vi "ConvertBase64StringToBytes.vi"(11 "Base64 string":string) -> (1 "error":bool, 3 "U8 array":u8[](array[numeric]))   [LabVIEW 2017]
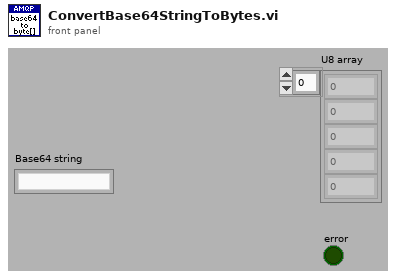
[diagram p1: front panel]
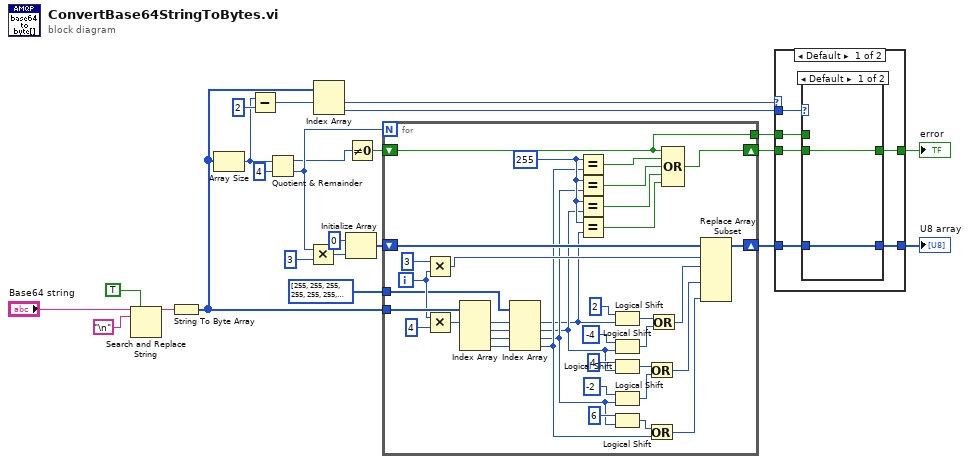
[diagram p0: block diagram]
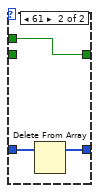
[diagram p2: hidden frame]
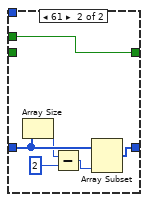
[diagram p3: hidden frame]
diagram:
  n1 = Search and Replace String(replace all?=TRUE ("replace all? (F)"), input string="Base64 string", search string="\n") -> (result string=w6:string)  [unwired: 1 in, 7 out]
  n2 = String To Byte Array(string=w6) -> (unsigned byte array=w9:u8[])
  n3 = Array Size(array=w9) -> (size(s)=w14:i32)
  n4 = Subtract(x=w14, y=2 ("x")) -> (x-y=w13:i32)
  n5 = Quotient & Remainder(x=w14, y=4) -> (x-y*floor(x/y)=w16:i32, floor(x/y)=w20:i32)
  n6 = Multiply(x=w20, y=3) -> (x*y=w19:i32)
  n7 = Index Array(array=w9, index #1=w13) -> (element #1=w12:u8, element #2=w11:u8)  [unwired: 1 in]
  n8 = Initialize Array(u8 0 ("Numeric"), w19) -> (w21:u8[])
  n9 = Not Equal To 0?(x=w16) -> (x != 0?=w8:bool)
  n10 = for {
    N: w20 -> [_]
    shift-right: [w57] -> w15
    shift-left: w21 -> [w58]
    tunnel: w9 -> [w61]
    tunnel: u8[] [255, 255, 255, 255, 255, 255, 255, 255, 255, 255, 255, 255, 255, 255, 255, 255, 255, 255, 255, 255, 255, 255, 255, 255, 255, 255, 255, 255, 255, 255, 255, 255, 255, 255, 255, 255, 255, 255, 255, 255, 255, 255, 255, 62, 255, 255, 255, 63, 52, 53, 54, 55, 56, 57, 58, 59, 60, 61, 255, 255, 255, 255, 255, 255, 255, 0, 1, 2, 3, 4, 5, 6, 7, 8, 9, 10, 11, 12, 13, 14, 15, 16, 17, 18, 19, 20, 21, 22, 23, 24, 25, 255, 255, 255, 255, 255, 255, 26, 27, 28, 29, 30, 31, 32, 33, 34, 35, 36, 37, 38, 39, 40, 41, 42, 43, 44, 45, 46, 47, 48, 49, 50, 51, 255, 255, 255, 255, 255, 255, 255, 255, 255, 255, 255, 255, 255, 255, 255, 255, 255, 255, 255, 255, 255, 255, 255, 255, 255, 255, 255, 255, 255, 255, 255, 255, 255, 255, 255, 255, 255, 255, 255, 255, 255, 255, 255, 255, 255, 255, 255, 255, 255, 255, 255, 255, 255, 255, 255, 255, 255, 255, 255, 255, 255, 255, 255, 255, 255, 255, 255, 255, 255, 255, 255, 255, 255, 255, 255, 255, 255, 255, 255, 255, 255, 255, 255, 255, 255, 255, 255, 255, 255, 255, 255, 255, 255, 255, 255, 255, 255, 255, 255, 255, 255, 255, 255, 255, 255, 255, 255, 255, 255, 255, 255, 255, 255, 255, 255, 255, 255, 255, 255, 255, 255, 255, 255, 255, 255, 255, 255, 255, 255, 255, 255, 255, 255] ("Array") -> [w43]
    shift-right: [w25] -> w2
    shift-left: w8 -> [w30]
    tunnel: [w30] -> w1
    i -> [w56]
    w35 = u8 255 ("x")
    n11 = Multiply(x=3, y=w56) -> (x*y=w54:i32)
    n12 = Multiply(x=w56, y=4 ("x")) -> (x*y=w59:i32)
    n13 = Index Array(array=w61, index #1=w59) -> (element #1=w42:u8, element #2=w41:u8, element #3=w40:u8, element #4=w39:u8)  [unwired: 3 in]
    n14 = Index Array(array=w43, index #1=w42, index #2=w41, index #3=w40, index #4=w39) -> (element #1=w26:u8, element #2=w27:u8, element #3=w28:u8, element #4=w29:u8)
    n15 = Equal?(x=w35, y=w29) -> (x = y?=w34:bool)
    n16 = Equal?(x=w35, y=w28) -> (x = y?=w33:bool)
    n17 = Equal?(x=w35, y=w27) -> (x = y?=w32:bool)
    n18 = Equal?(x=w35, y=w26) -> (x = y?=w31:bool)
    n19 = Logical Shift(y=i8 2, x=w26) -> (x << y=w50:u8)
    n20 = Logical Shift(y=i8 -4, x=w27) -> (x << y=w49:u8)
    n21 = Logical Shift(y=i8 4, x=w27) -> (x << y=w52:u8)
    n22 = Logical Shift(y=i8 -2, x=w28) -> (x << y=w51:u8)
    n23 = Logical Shift(y=i8 6, x=w28) -> (x << y=w53:u8)
    n24 = Or(x=w52, y=w51) -> (x .or. y?=w37:u8)
    n25 = Or(x=w53, y=w29) -> (x .or. y?=w36:u8)
    n26 = Or(x=w50, y=w49) -> (x .or. y?=w38:u8)
    n27 = Compound Arithmetic op=OR(w30, w34, w33, w32, w31) -> (w25:bool)
    n28 = Replace Array Subset(array=w58, new element #1=w38, index #1=w54, new element #2=w37, new element #3=w36) -> (w57:u8[])  [unwired: 2 in]
  }
  n29 = case shown="Default" w12 {
    tunnel: [w66 w78] -> w10
    tunnel: w15 -> [w67 w77]
    tunnel: w11 -> [w65 _]
    tunnel: [w64 w73] -> w3
    tunnel: w2 -> [w63 _]
    tunnel: w1 -> [w62 w73]
    frame Default {
      n30 = case shown="Default" w65 {
        tunnel: w67 -> [w69 w72]
        tunnel: [w69 w71] -> w66
        tunnel: [w68 w70] -> w64
        tunnel: w63 -> [w68 _]
        tunnel: w62 -> [_ w70]
        frame Default {
        }
        frame 61 {
          n31 = Delete From Array(array=w72) -> (array with subset deleted=w71:u8[])  [unwired: 2 in, 1 out]
        }
      }
    }
    frame 61 {
      n32 = Array Size(array=w77) -> (size(s)=w76:i32)
      n33 = Subtract(x=w76, y=2) -> (x-y=w74:i32)
      n34 = Array Subset(array=w77, length=w74) -> (w78:u8[])  [unwired: 1 in]
    }
  }
  "U8 array" <- w10
  "error" <- w3
